vi "ReadFPGAandPublishMQTT.vi"(8 "error in (no error)":errorcluster, 10 "FPGA VI Reference":T1, 11 "MQTT":refnum<k5>) -> (0 "error out":errorcluster, 3 "connection ID out":refnum<k5>)   [LabVIEW 2024]
uses:
  FPGA VI Ref.ctl
  <vilib>/Utility/error.llb/Error Cluster From Error Code.vi
  <vilib>/rvi/errors/niLvFpgaAdjustHostInterfaceError.vi
  <vilib>/rvi/interface/nirviReadWriteControl/nirviReadWriteControl.xnode
  LVMQTT-master/MQTT_Functions.lvlib
  NiFpgaLv.dll
  <vilib>/rvi/interface/Simulation/niFpgaSimulationCallBeginRW.vi
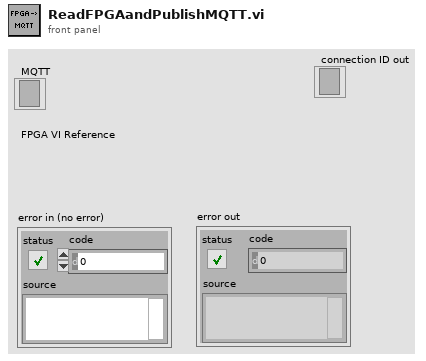
[diagram p1: front panel]
types:
  T1 = typedef "FPGA VI Ref.ctl" = refnum<k20>
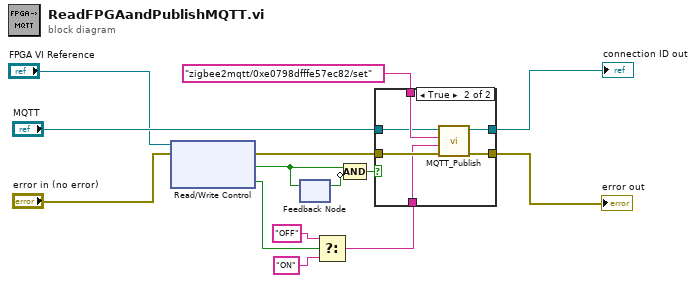
[diagram p0: block diagram]
diagram:
  n1 = xnode "Read/Write Control"("FPGA VI Reference In"="FPGA VI Reference", "error in"="error in (no error)") -> ("error out"=w9:errorcluster, "Kiuas Switch"=w13:bool, "Kiuas LED"=w5:bool)  [unwired: 1 out]
  n2 = feedback-in #1(w13) -> ()
  n3 = feedback #1() -> (w14:bool)  [unwired: 1 in]
  n4 = Select(t="OFF" ("Topic"), s=w5, f="ON" ("Topic")) -> (s? t:f=w2:string)
  n5 = Compound Arithmetic op=AND(w13, invert w14) -> (w6:bool)
  n6 = case shown="True" w6 {
    tunnel: "zigbee2mqtt/0xe0798dfffe57ec82/set" ("Topic") -> [_ w22]
    tunnel: "MQTT" -> [w16 w21]
    tunnel: w9 -> [w15 w20]
    tunnel: [w15 w17] -> w8
    tunnel: [w16 w18] -> w7
    tunnel: w2 -> [_ w19]
    frame False {
    }
    frame True {
      n7 = call "MQTT_Publish.vi"("error in (no error)"=w20, "Message to be published"=w19, "Topic"=w22, "connection ID"=w21) -> ("error out"=w17:errorcluster, "connection ID out"=w18:refnum<k5>)  [unwired: 6 in]
    }
  }
  "error out" <- w8
  "connection ID out" <- w7
